vi "KE622x -- 2182 -A Set Digital Filter State.vi"(0 "622x Resource In":refnum<visa-resource-name>, 1 "Check For SCPI Errors? (T)":bool=TRUE, 7 "Enable Digital Filter?":bool, 11 "error in (no error)":errorcluster) -> (4 "622x Resource Out (dupl)":refnum<visa-resource-name>, 15 "error out":errorcluster)   [LabVIEW 2019, in "Keithley 622x.lvlib"]
uses:
  Keithley 622x.lvlib
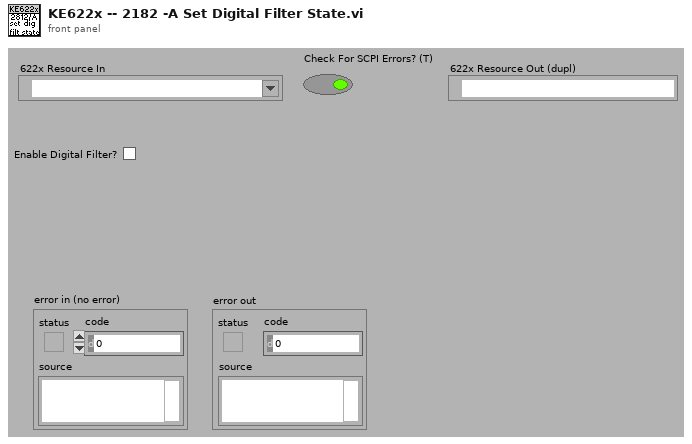
[diagram p1: front panel]
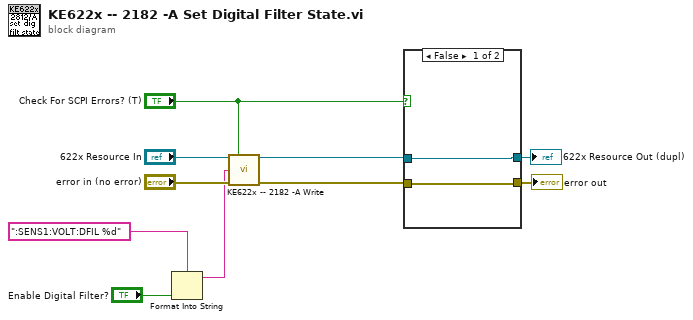
[diagram p0: block diagram]
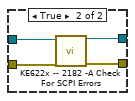
[diagram p2: hidden frame]
diagram:
  n1 = Format Into String(format string=":SENS1:VOLT:DFIL %d", "Enable Digital Filter?") -> (resulting string=w3:string)  [unwired: 2 in, 1 out]
  n2 = call "KE622x -- 2182 -A Write.vi"("Resource In"="622x Resource In", "Check For SCPI Errors? (T)"="Check For SCPI Errors? (T)", "2182-A Write String"=w3, "error in (no error)"="error in (no error)") -> ("Resource Out (dupl)"=w8:refnum<visa-resource-name>, "error out"=w2:errorcluster)  [unwired: 10 in]
  n3 = case shown="False" "Check For SCPI Errors? (T)" {
    tunnel: w8 -> [w12 w16]
    tunnel: w2 -> [w11 w15]
    tunnel: [w12 w14] -> w6
    tunnel: [w11 w13] -> w5
    frame False {
    }
    frame True {
      n4 = call "KE622x -- 2182 -A Check For SCPI Errors.vi"("VISA Resource In"=w16, "error in (no error)"=w15) -> ("VISA Resource Out (dupl)"=w14:refnum<visa-resource-name>, "error out"=w13:errorcluster)  [unwired: 10 in, 2 out]
    }
  }
  "622x Resource Out (dupl)" <- w6
  "error out" <- w5
